vi "Folder Structure.vi"(8 "error in (no error)":errorcluster, 11 "folder structure  to create if nonexistant":path) -> (0 "error out":errorcluster, 1 "structure created":bool, 2 "status string":string, 3 "directory (dup)":path)   [LabVIEW 2020]
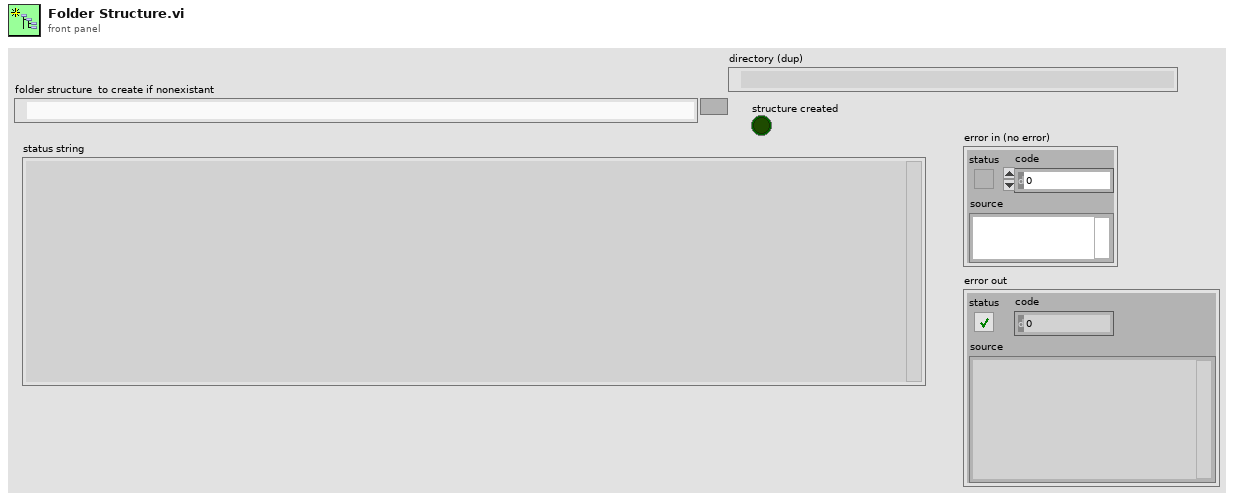
[diagram p1: front panel]
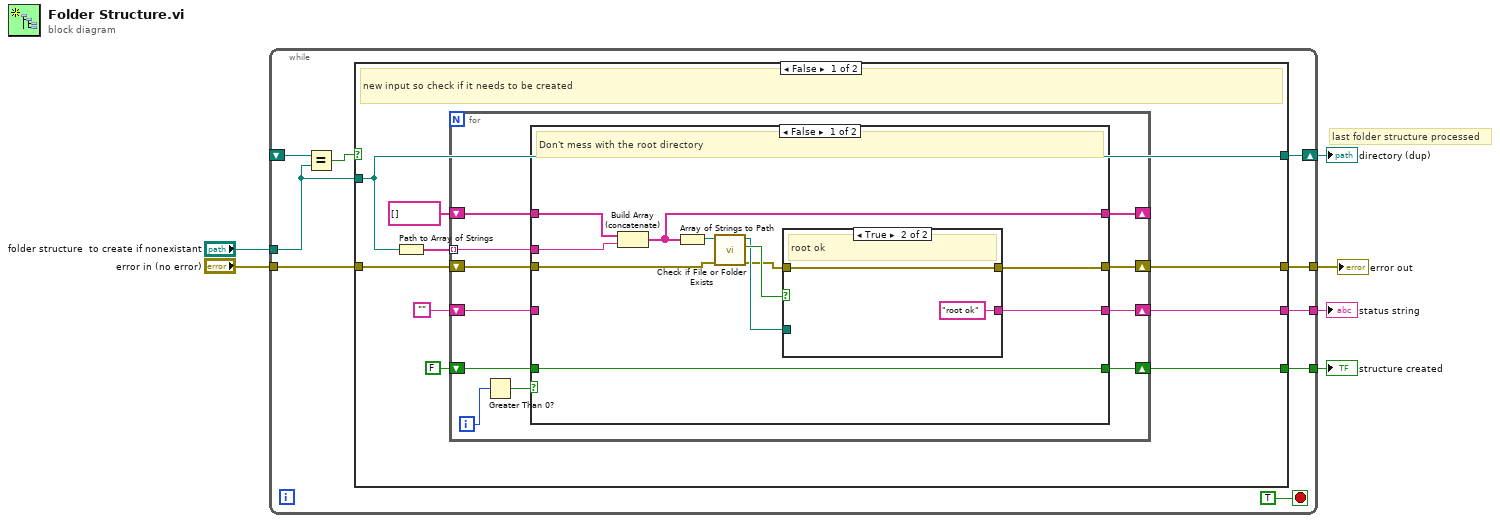
[diagram p0: block diagram]
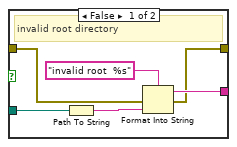
[diagram p2: hidden frame]
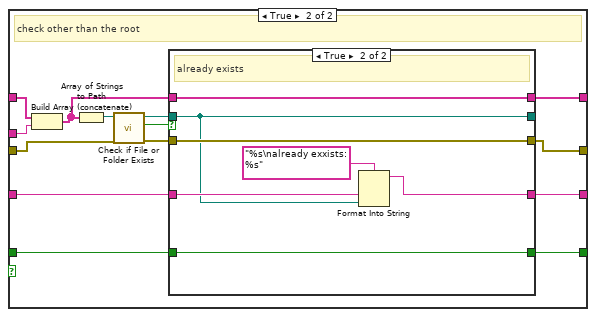
[diagram p3: hidden frame]
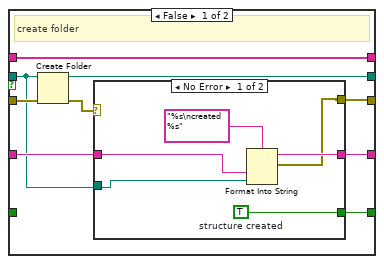
[diagram p4: hidden frame]
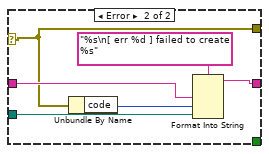
[diagram p5: hidden frame]
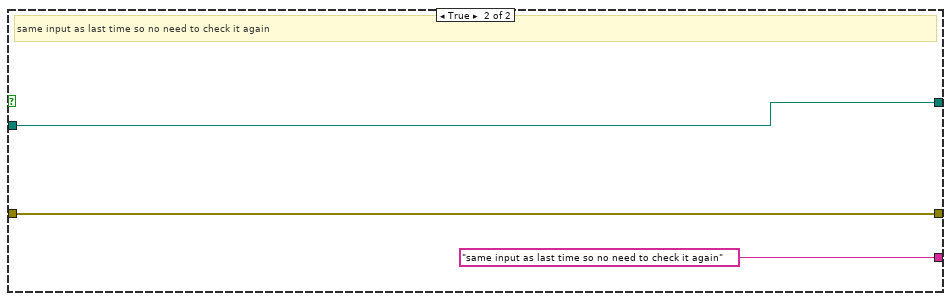
[diagram p6: hidden frame]
diagram:
  # "last folder structure processed"
  n1 = while {
    tunnel: "folder structure  to create if nonexistant" -> [w8]
    shift-right: [w15] -> w2
    shift-left: _ -> [w14]
    tunnel: "error in (no error)" -> [w12]
    tunnel: [w10] -> w4
    tunnel: [w9] -> w3
    tunnel: [w7] -> w1
    stop <- TRUE stop-if-true
    n2 = Equal?(x=w14, y=w8) -> (x = y?=w13:bool)
    n3 = case shown="False" w13 {
      tunnel: [w18 w98] -> w15
      tunnel: w12 -> [w22 w99]
      tunnel: [w19 w99] -> w10
      tunnel: [w20 "same input as last time so no need to check it again"] -> w9
      tunnel: w8 -> [w18 w98]
      tunnel: [w17 _] -> w7
      frame False {
        # "new input so check if it needs to be created"
        n4 = Path to Array of Strings(0:w18) -> (2:w24:string[])  [unwired: 1 out]
        n5 = for {
          tunnel: w24 -> [w33] mode=indexing
          shift-right: [w31] -> _
          shift-left: string[] [] -> [w32]
          shift-right: [w29] -> w19
          shift-left: w22 -> [w30]
          shift-right: [w28] -> w20
          shift-left: "" -> [w27]
          shift-right: [w26] -> w17
          shift-left: FALSE ("structure created") -> [w25]
          i -> [w35]
          n6 = Greater Than 0?(x=w35) -> (x > 0?=w34:bool)
          n7 = case shown="False" w34 {
            tunnel: w33 -> [w45 w64]
            tunnel: w32 -> [w46 w63]
            tunnel: [w43 w59] -> w31
            tunnel: w30 -> [w42 w62]
            tunnel: [w37 w61] -> w29
            tunnel: [w38 w58] -> w28
            tunnel: w27 -> [_ w57]
            tunnel: [w36 w56] -> w26
            tunnel: w25 -> [w36 w55]
            frame False {
              # "Don't mess with the root directory"
              n8 = Build Array (concatenate)(w46, w45) -> (w43:string[])
              n9 = Array of Strings to Path(0:w43) -> (2:w44:path)  [unwired: 1 in]
              n10 = call <vilib>:"Check if File or Folder Exists.vi"("error in (no error)"=w42, "path"=w44) -> ("error out"=w39:errorcluster, "file or folder exists?"=w41:bool, "dup path"=w40:path)  [unwired: 7 in]
              n11 = case shown="True" w41 {
                tunnel: w40 -> [w51 _]
                tunnel: w39 -> [w50 w54]
                tunnel: [w49 "root ok"] -> w38
                tunnel: [w48 w54] -> w37
                frame False {
                  # "invalid root directory"
                  n12 = Path To String(path=w51) -> (string=w47:string)
                  n13 = Format Into String(format string="invalid root  %s", error in=w50, w47) -> (resulting string=w49:string, error out=w48:errorcluster)  [unwired: 1 in]
                }
                frame True {
                  # "root ok"
                }
              }
            }
            frame True {
              # "check other than the root"
              n14 = Build Array (concatenate)(w63, w64) -> (w60:string[])
              n15 = Array of Strings to Path(0:w60) -> (2:w68:path)  [unwired: 1 in]
              n16 = call <vilib>:"Check if File or Folder Exists.vi"("error in (no error)"=w62, "path"=w68) -> ("error out"=w65:errorcluster, "file or folder exists?"=w67:bool, "dup path"=w66:path)  [unwired: 7 in]
              n17 = case shown="True" w67 {
                tunnel: w66 -> [w71 w91]
                tunnel: w65 -> [w77 w96]
                tunnel: [w70 w96] -> w61
                tunnel: [w76 w91] -> _
                tunnel: w60 -> [w75 w95]
                tunnel: [w75 w95] -> w59
                tunnel: [w73 w92] -> w58
                tunnel: w57 -> [w72 w93]
                tunnel: [w69 w90] -> w56
                tunnel: w55 -> [_ w90]
                frame False {
                  # "create folder"
                  n18 = Create Folder(path (use dialog)=w71, error in=w77) -> (created path=w76:path, error out=w74:errorcluster)  [unwired: 1 in, 1 out]
                  n19 = case shown="No Error" w74 {
                    selector: w74 -> [_ w84]
                    tunnel: [w82 w85] -> w73
                    tunnel: w72 -> [w81 w88]
                    tunnel: w71 -> [w80 w86]
                    tunnel: [w79 w84] -> w70
                    tunnel: [w78 _] -> w69
                    frame No Error {
                      w78 = TRUE  # structure created
                      n20 = Format Into String(format string="%s\ncreated %s", w81, w80) -> (resulting string=w82:string, error out=w79:errorcluster)  [unwired: 2 in]
                    }
                    frame Error {
                      n21 = Unbundle By Name(w84) -> ("code"=w87:i32)
                      n22 = Format Into String(format string="%s\n[ err %d ] failed to create %s", w88, w87, w86) -> (resulting string=w85:string)  [unwired: 2 in, 1 out]
                    }
                  }
                }
                frame True {
                  # "already exists"
                  n23 = Format Into String(format string="%s\nalready exxists:  %s", w93, w91) -> (resulting string=w92:string)  [unwired: 2 in, 1 out]
                }
              }
            }
          }
        }
      }
      frame True {
        # "same input as last time so no need to check it again"
      }
    }
  }
  "error out" <- w4
  "status string" <- w3
  "directory (dup)" <- w2
  "structure created" <- w1
